vi "Day 5.vi"() -> ()   [LabVIEW 2020]
uses:
  <userlib>/_OpenG.lib/array/array.llb/Conditional Auto-Indexing Tunnel (U32)__ogtk.vi
panel:
  out "Numeric":u32
  out "element":string
  out "max value":u32
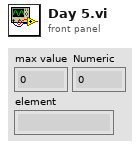
[diagram p1: front panel]
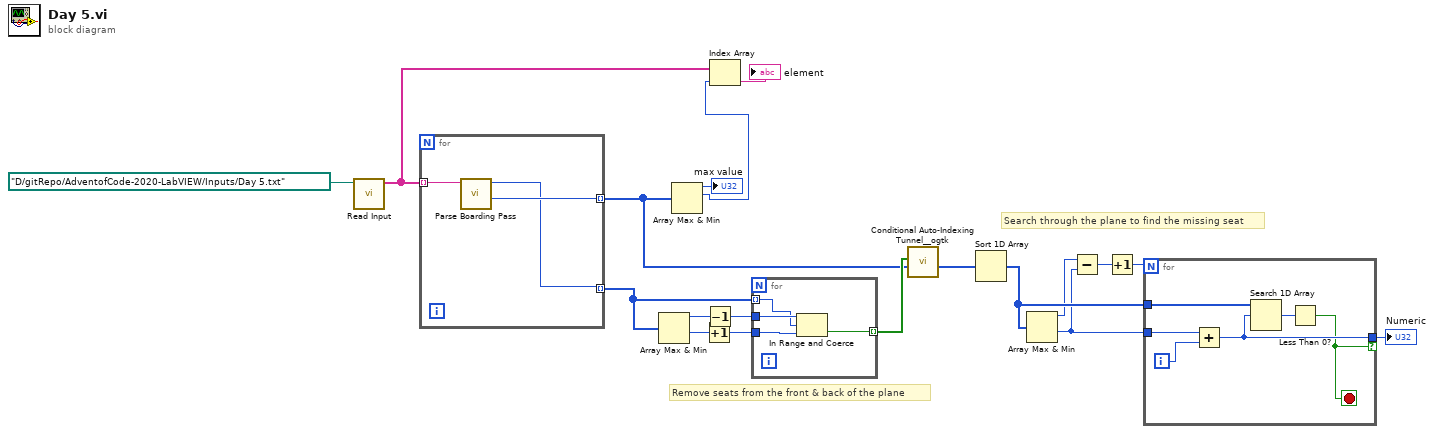
[diagram p0: block diagram]
diagram:
  # "Search through the plane to find the missing seat"
  # "Remove seats from the front & back of the plane"
  n1 = call "Read Input.vi"("Path"=path "D:/gitRepo/AdventofCode-2020-LabVIEW/Inputs/Day 5.txt") -> ("string array"=w17:string[])  [unwired: 10 in]
  n2 = for {
    tunnel: w17 -> [w22] mode=indexing
    tunnel: [w21] -> w9 mode=indexing
    tunnel: [w20] -> w8 mode=indexing
    n3 = call "Parse Boarding Pass.vi"("Boarding Pass"=w22) -> ("Seat ID"=w21:u32, "Row"=w20:u32)  [unwired: 8 in, 1 out]
  }
  n4 = Array Max & Min(array=w8) -> (max value=w14:u32, min value=w13:u32)  [unwired: 2 out]
  n5 = Array Max & Min(array=w9) -> (max value=→"max value":u32, max index (indices)=w16:i32)  [unwired: 2 out]
  n6 = Increment(x=w13) -> (x+1=w11:u32)
  n7 = Decrement(x=w14) -> (x-1=w12:u32)
  n8 = Index Array(array=w17, index=w16) -> (element=→"element":string)
  n9 = for {
    tunnel: w12 -> [w26]
    tunnel: w11 -> [w25]
    tunnel: [w24] -> w10 mode=indexing
    tunnel: w8 -> [w23] mode=indexing
    n10 = In Range and Coerce(upper limit=w26, x=w23, lower limit=w25) -> (In Range?=w24:bool)  [unwired: 1 out]
  }
  n11 = call-poly <userlib>:"Conditional Auto-Indexing Tunnel__ogtk.vi"("Array in"=w9, "Elements to keep"=w10) -> ("Filtered Array out"=w7:u32[])  [unwired: 5 in]
  n12 = Sort 1D Array(array=w7) -> (sorted array=w6:u32[])
  n13 = Array Max & Min(array=w6) -> (max value=w5:u32, min value=w2:u32)  [unwired: 2 out]
  n14 = Subtract(x=w5, y=w2) -> (x-y=w4:u32)
  n15 = Increment(x=w4) -> (x+1=w3:u32)
  n16 = for {
    N: w3 -> [_]
    tunnel: w6 -> [w32]
    tunnel: w2 -> [w31]
    tunnel: [w28] -> w1 if=w27
    i -> [w30]
    stop <- w27 stop-if-true
    n17 = Add(x=w31, y=w30) -> (x+y=w28:u32)
    n18 = Search 1D Array(1D array=w32, element=w28) -> (index of element=w29:i32)  [unwired: 1 in]
    n19 = Less Than 0?(x=w29) -> (x < 0?=w27:bool)
  }
  "Numeric" <- w1
